vi "Labview_USB_SPI_SlaveTest.vi"() -> ()   [LabVIEW 2010]
uses:
  <userlib>/Ginkgo_Driver/Ginkgo_Driver.dll
panel:
  out "error out":errorcluster
  in  "stop":bool
  in  "OK":bool
  out "Read Data Num":dbl
  in  "LSBFirst":u16(ring) items=["0", "1"]
  in  "CPHA":u16(ring) items=["0", "1"]
  in  "CPOL":u16(ring) items=["0", "1"]
  in  "Append/Replace":bool
  out "Read Data(Hex)":string
  in  "Channel Index":u16(ring) items=["0", "1"]
  in  "Device Index":u16(ring) items=["0", "1", "2", "3", "4", "5", "6", "7", "8", "9"]
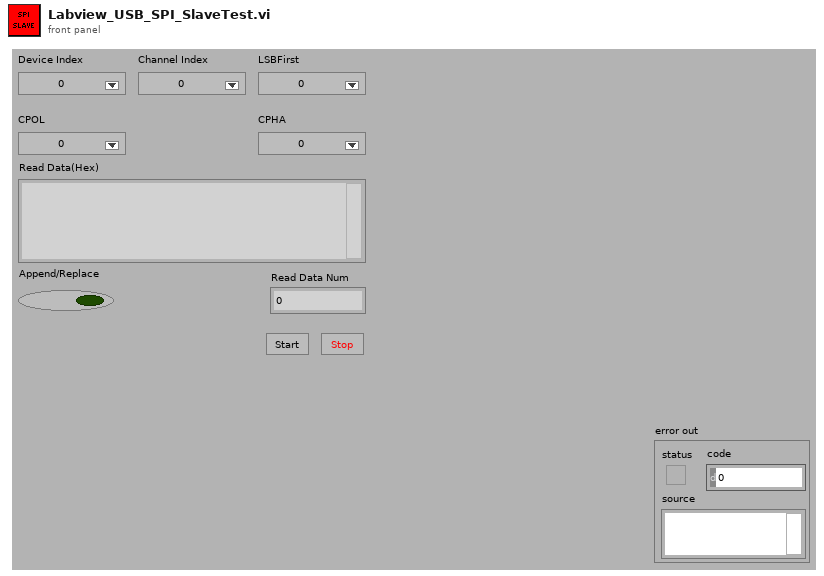
[diagram p1: front panel]
types:
  T1 = enum16{"Init", "ScanDevice", "OpenDevice", "InitDevice", "Read data", "Idel", "Error"}
  T2 = cluster{"ControlMode":u8, "TranBits":u8, "MasterMode":u8, "CPOL":u8, "CPHA":u8, "LSBFirst":u8, "SelPolarity":u8, "@dummy control@":i8, "ClockSpeed":u32}
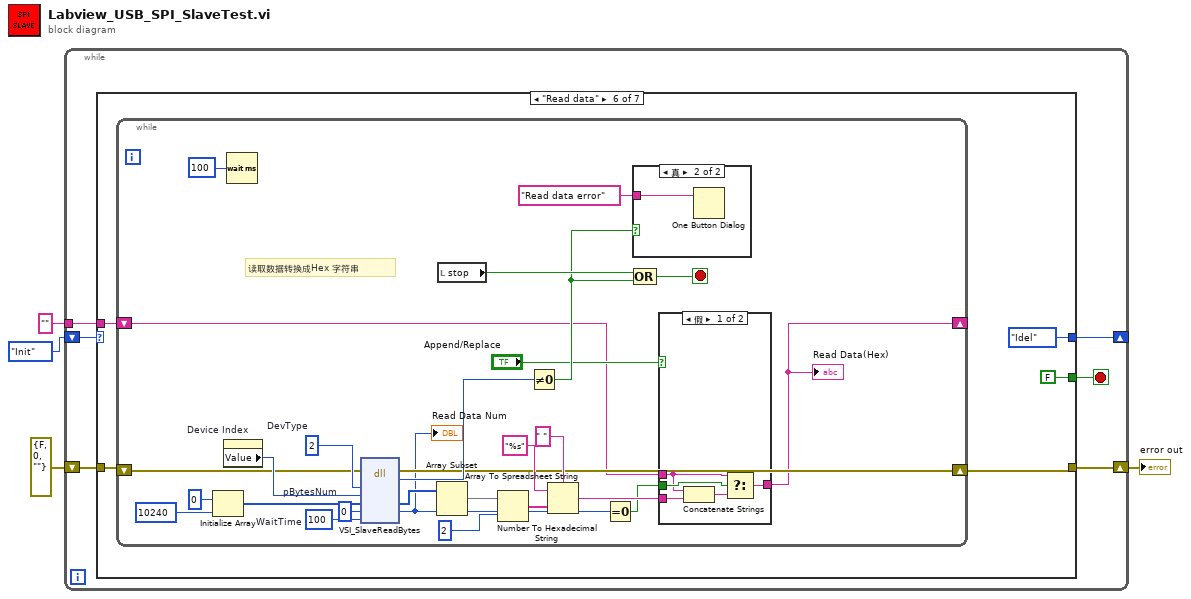
[diagram p0: block diagram]
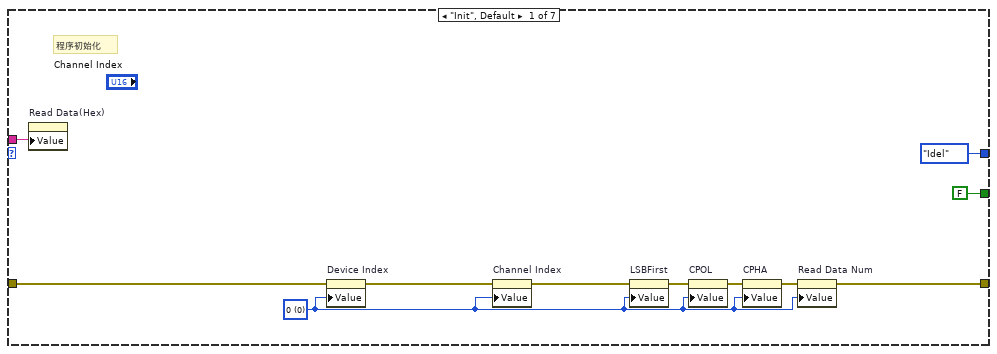
[diagram p2: hidden frame]
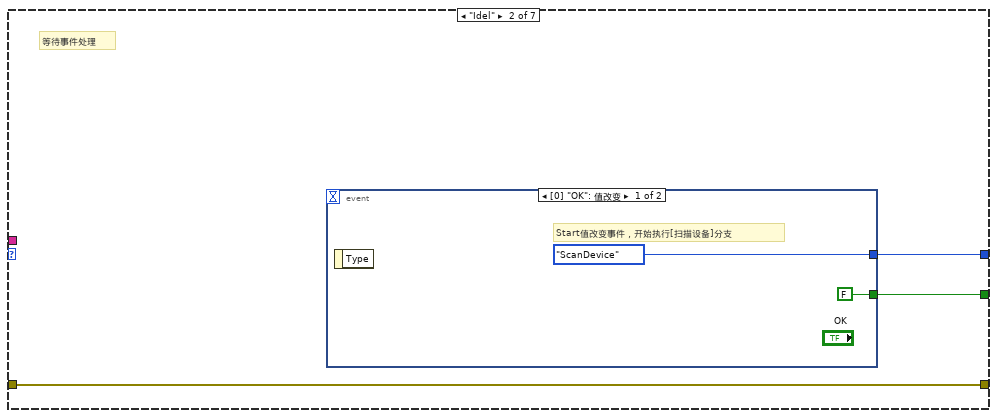
[diagram p3: hidden frame]
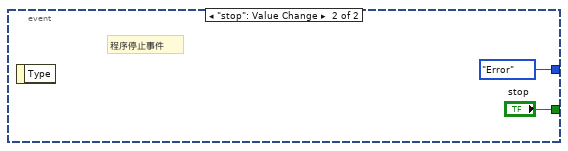
[diagram p4: hidden frame]
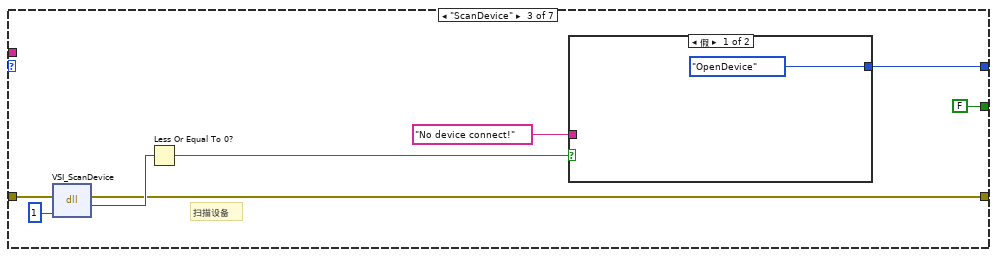
[diagram p5: hidden frame]
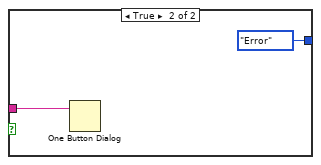
[diagram p6: hidden frame]
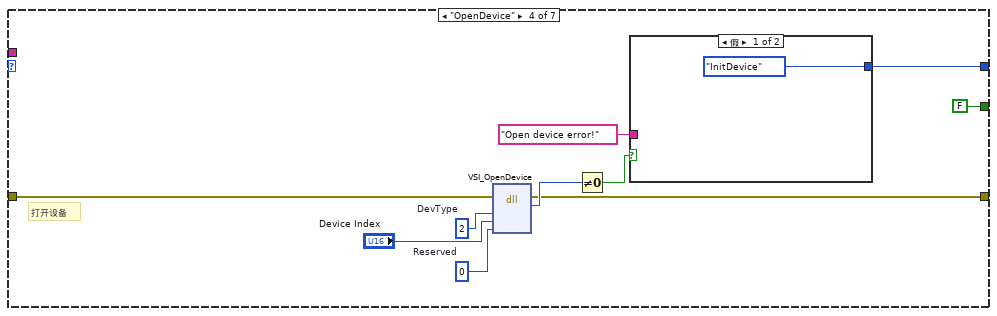
[diagram p7: hidden frame]
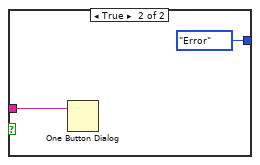
[diagram p8: hidden frame]
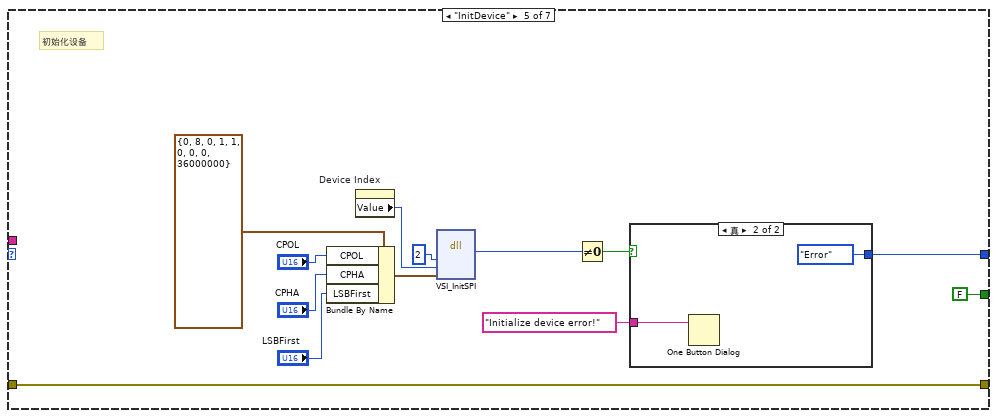
[diagram p9: hidden frame]
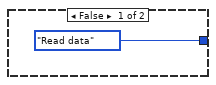
[diagram p10: hidden frame]
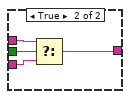
[diagram p11: hidden frame]
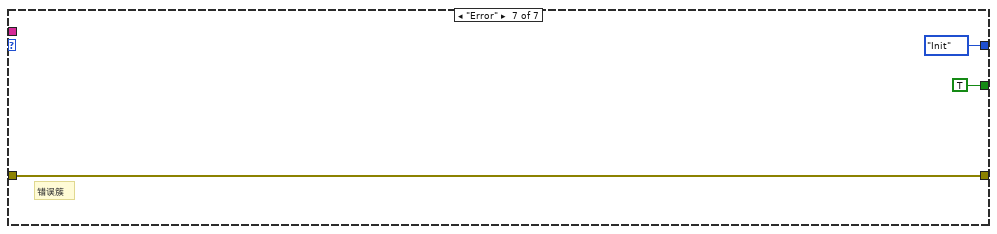
[diagram p13: hidden frame]
diagram:
  n1 = while {
    shift-right: [w10] -> _
    shift-left: T1."Init" ("Enum") -> [w9]
    shift-right: [w7] -> w2
    shift-left: errorcluster {"status"=FALSE, "code"=0, "source"=""} ("error out") -> [w6]
    tunnel: "" ("Read Data(Hex)") -> [w5]
    stop <- w8 stop-if-true
    n2 = case shown="\"Read data\"" w9 {
      tunnel: [T1."Idel" ("Enum") w23 w32 w43 w60 T1."Idel" ("Enum") T1."Init" ("Enum")] -> w10
      tunnel: [FALSE ("stop") w24 FALSE ("stop") FALSE ("stop") FALSE ("stop") FALSE ("stop") TRUE ("stop")] -> w8
      tunnel: [w12 w22 w30 w40 w53 w69 w111] -> w7
      tunnel: w6 -> [w13 w22 w29 w41 w53 w70 w111]
      tunnel: w5 -> [w11 _ _ _ _ w71 _]
      frame "Init", Default {
        w19 = u16 0 items=["0", "1", "2", "3", "4", "5", "6", "7", "8", "9"] ("Device Index")
        # "程序初始化"
        n3 = property on="Read Data(Hex)" class="Str"("Value"=w11) -> ()  [unwired: 2 in, 2 out]
        n4 = property on="Device Index" class="Ring (严格)"(error in=w13, "Value"=w19) -> (error out=w18:errorcluster)  [unwired: 1 in, 1 out]
        n5 = property on="Channel Index" class="Ring (严格)"(error in=w18, "Value"=w19) -> (error out=w17:errorcluster)  [unwired: 1 in, 1 out]
        n6 = property on="LSBFirst" class="Ring (严格)"(error in=w17, "Value"=w19) -> (error out=w16:errorcluster)  [unwired: 1 in, 1 out]
        n7 = property on="CPOL" class="Ring (严格)"(error in=w16, "Value"=w19) -> (error out=w15:errorcluster)  [unwired: 1 in, 1 out]
        n8 = property on="CPHA" class="Ring (严格)"(error in=w15, "Value"=w19) -> (error out=w14:errorcluster)  [unwired: 1 in, 1 out]
        n9 = property on="Read Data Num" class="DigNum (严格)"(error in=w14, "Value"=w19) -> (error out=w12:errorcluster)  [unwired: 1 in, 1 out]
      }
      frame "Idel" {
        # "等待事件处理"
        n10 = event shown="[0] \"OK\": 值改变" {
          selector: _ -> [_ _]
          dyn-events: _ -> [_ _]
          timeout: _ -> [_ _]
          tunnel: [FALSE ("stop") "stop"] -> w24
          tunnel: [T1."ScanDevice" ("Enum") T1."Error" ("Enum")] -> w23
          event "OK": Value Change {
            # "Start值改变事件，开始执行[扫描设备]分支"
            n11 = event-data() -> ()  [unwired: 1 in, 1 out]
          }
          event "stop": Value Change {
            # "程序停止事件"
            n12 = event-data() -> ()  [unwired: 1 in, 1 out]
          }
        }
      }
      frame "ScanDevice" {
        # "扫描设备"
        n13 = dll-call lib="D:/Program Files (x86)/National Instruments/LabVIEW 2010/user.lib/Ginkgo_Driver/Ginkgo_Driver.*" fn="VSI_ScanDevice"(error in=w29, "NeedInit"=u8 1) -> (error out=w30:errorcluster, "return type"=w35:i32)  [unwired: 3 in, 1 out]
        n14 = Less Or Equal To 0?(x=w35) -> (x <= 0?=w34:bool)
        n15 = case shown="假" w34 {
          tunnel: "No device connect!" ("message") -> [_ w39]
          tunnel: [T1."OpenDevice" ("Enum") T1."Error" ("Enum")] -> w32
          frame False {
          }
          frame True {
            n16 = One Button Dialog(message=w39) -> ()  [unwired: 1 in, 1 out]
          }
        }
      }
      frame "OpenDevice" {
        w48 = 0  # Reserved
        w49 = 2  # DevType
        # "打开设备"
        n17 = dll-call lib="D:/Program Files (x86)/National Instruments/LabVIEW 2010/user.lib/Ginkgo_Driver/Ginkgo_Driver.*" fn="VSI_OpenDevice"(error in=w41, "DevType"=w49, "DevIndex"="Device Index", "Reserved"=w48) -> (error out=w40:errorcluster, w45:i32)  [unwired: 5 in, 1 out]
        n18 = Not Equal To 0?(x=w45) -> (x != 0?=w44:bool)
        n19 = case shown="假" w44 {
          tunnel: "Open device error!" ("message") -> [_ w52]
          tunnel: [T1."InitDevice" ("Enum") T1."Error" ("Enum")] -> w43
          frame False {
          }
          frame True {
            n20 = One Button Dialog(message=w52) -> ()  [unwired: 1 in, 1 out]
          }
        }
      }
      frame "InitDevice" {
        # "初始化设备"
        n21 = Bundle By Name(cluster=T2 {"ControlMode"=0, "TranBits"=8, "MasterMode"=0, "CPOL"=1, "CPHA"=1, "LSBFirst"=0, "SelPolarity"=0, "@dummy control@"=0, "ClockSpeed"=36000000} ("pInitConfig"), "CPOL"="CPOL", "CPHA"="CPHA", "LSBFirst"="LSBFirst") -> (w58:T2)
        n22 = property on="Device Index" class="Ring (严格)"() -> ("Value"=w64:u16)  [unwired: 2 in, 2 out]
        n23 = dll-call lib="D:/Program Files (x86)/National Instruments/LabVIEW 2010/user.lib/Ginkgo_Driver/Ginkgo_Driver.*" fn="VSI_InitSPI"("DevType"=2, "DevIndex"=w64, "pInitConfig"=w58) -> (w62:i32)  [unwired: 6 in, 2 out]
        n24 = Not Equal To 0?(x=w62) -> (x != 0?=w61:bool)
        n25 = case shown="真" w61 {
          tunnel: "Initialize device error!" ("message") -> [_ w68]
          tunnel: [T1."Read data" ("Enum") T1."Error" ("Enum")] -> w60
          frame False {
          }
          frame True {
            n26 = One Button Dialog(message=w68) -> ()  [unwired: 1 in, 1 out]
          }
        }
      }
      frame "Read data" {
        n27 = while {
          shift-right: [w74] -> _
          shift-left: w71 -> [w78]
          shift-right: [w80] -> w69
          shift-left: w70 -> [w81]
          stop <- w92 stop-if-true
          w100 = 2  # DevType
          w95 = 100  # WaitTime
          w96 = 0  # pBytesNum
          # "读取数据转换成Hex 字符串"
          n28 = Initialize Array(u8 0 ("元素"), 10240 ("维数大小")) -> (w99:u8[])
          n29 = property on="Device Index" class="Ring (严格)"() -> ("Value"=w93:u16)  [unwired: 2 in, 2 out]
          n30 = Wait (ms)(milliseconds to wait=u32 100) -> ()  [unwired: 1 out]
          n31 = dll-call lib="D:/Program Files (x86)/National Instruments/LabVIEW 2010/user.lib/Ginkgo_Driver/Ginkgo_Driver.*" fn="VSI_SlaveReadBytes"(error in=w81, "DevType"=w100, "DevIndex"=w93, "pReadData"=w99, "pBytesNum"=w96, "WaitTime"=w95) -> (error out=w80:errorcluster, w94:i32, "pReadData"=w85:u8[], "pBytesNum"=w76:i32)  [unwired: 5 in, 1 out]
          "Read Data Num" <- w76
          n32 = Array Subset(array=w85, length=w76) -> (w83:u8[])  [unwired: 1 in]
          n33 = local read "stop"() -> (w89:bool)
          n34 = Number To Hexadecimal String(1:i16 2 ("width (-)"), 2:w83) -> (0:w82:string[])
          n35 = Not Equal To 0?(x=w94) -> (x != 0?=w88:bool)
          n36 = Array To Spreadsheet String(delimiter (Tab)=" ", array=w82, 3:"%s" ("format string")) -> (spreadsheet string=w77:string)
          n37 = Equal To 0?(x=w76) -> (x = 0?=w75:bool)
          n38 = case shown="真" w88 {
            tunnel: "Read data error" ("message") -> [_ w110]
            frame False {
            }
            frame True {
              n39 = One Button Dialog(message=w110) -> ()  [unwired: 1 in, 1 out]
            }
          }
          n40 = Compound Arithmetic op=OR(w89, w88) -> (w92:bool)
          n41 = case shown="假" "Append/Replace" {
            tunnel: w78 -> [w103 w109]
            tunnel: w77 -> [w102 w108]
            tunnel: [w101 w107] -> w74
            tunnel: w75 -> [w105 w106]
            frame False {
              n42 = Concatenate Strings(w103, w102) -> (w104:string)
              n43 = Select(t=w103, s=w105, f=w104) -> (s? t:f=w101:string)
            }
            frame True {
              n44 = Select(t=w109, s=w106, f=w108) -> (s? t:f=w107:string)
            }
          }
          "Read Data(Hex)" <- w74
        }
      }
      frame "Error" {
        # "错误簇"
      }
    }
  }
  "error out" <- w2
